vi "GetPositionCOM.vi"(8 "error in":errorcluster, 9 "Axis":enum16{"X", "Y", "Z"}(ring), 11 "VISA resource name":refnum<visa-resource-name>) -> (0 "error out":errorcluster, 2 "Position (mm)":dbl, 3 "VISA resource name out":refnum<visa-resource-name>)   [LabVIEW 2017]
panel:
  out "Raw output (hex)":string
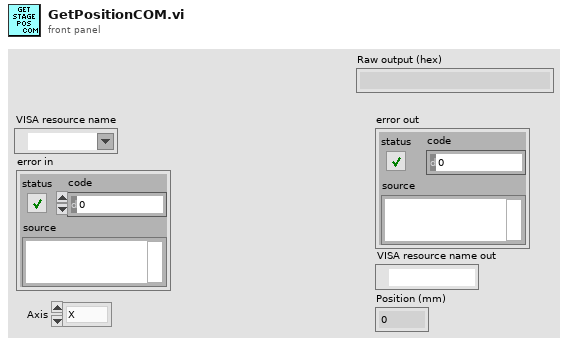
[diagram p1: front panel]
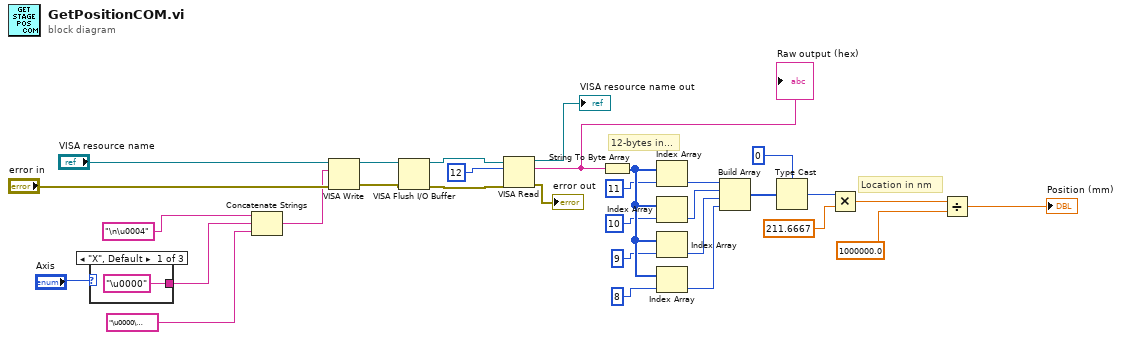
[diagram p0: block diagram]
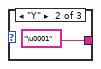
[diagram p2: hidden frame]
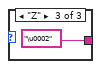
[diagram p3: hidden frame]
diagram:
  # "Location in nm"
  # "12-bytes in..."
  n1 = case shown="\"X\", Default" "Axis" {
    tunnel: ["\u0000" "\u0001" "\u0002"] -> w27
    frame "X", Default {
    }
    frame "Y" {
    }
    frame "Z" {
    }
  }
  n2 = Concatenate Strings("\n\u0004", w27, "\u0000\u0000\u0000") -> (w25:string)
  n3 = VISA Write(VISA resource name="VISA resource name", write buffer=w25, error in (no error)="error in") -> (VISA resource name out=w1:refnum<visa-resource-name>, error out=w4:errorcluster)  [unwired: 1 out]
  n4 = VISA Flush I/O Buffer(VISA resource name=w1, error in (no error)=w4) -> (VISA resource name out=w2:refnum<visa-resource-name>, error out=w3:errorcluster)  [unwired: 1 in]
  n5 = VISA Read(VISA resource name=w2, byte count=u32 12, error in (no error)=w3) -> (VISA resource name out=→"VISA resource name out":refnum<visa-resource-name>, read buffer=w24:string, error out=→"error out":errorcluster)  [unwired: 1 out]
  "Raw output (hex)" <- w24
  n6 = String To Byte Array(string=w24) -> (unsigned byte array=w23:u8[])
  n7 = Index Array(array=w23, index=11) -> (element=w18:u8)
  n8 = Index Array(array=w23, index=10) -> (element=w17:u8)
  n9 = Index Array(array=w23, index=9) -> (element=w16:u8)
  n10 = Index Array(array=w23, index=8) -> (element=w15:u8)
  n11 = Build Array(w18, w17, w16, w15) -> (w14:u8[])
  n12 = Type Cast(type=0 ("byte count"), x=w14) -> (*(type *) &x=w10:i32)
  n13 = Multiply(x=w10, y=211.6667) -> (x*y=w8:dbl)
  n14 = Divide(x=w8, y=1000000.0) -> (x/y=→"Position (mm)":dbl)
